vi "auto.vi"(11 "Inputs 2":T3) -> (3 "Outputs":T6)   [LabVIEW 2013]
uses:
  outputs.ctl
  drive/drive_outputs.ctl
  flinger/flinger_outputs.ctl
  <vilib>/Rock Robotics/WPI/Solenoid/WPI_SolenoidValue.ctl
  roller/roller_outputs.ctl
  catch/catch_outputs.ctl
  inputs.ctl
  drive/drive_inputs.ctl
  flinger/flinger_inputs.ctl
  roller/roller_inputs.ctl
  catch/catch_inputs.ctl
panel:
  in  "Flinger Inputs":T1
  in  "Roller Inputs":T2
  in  "Drive_inputs":T4
  in  "Inputs":T3
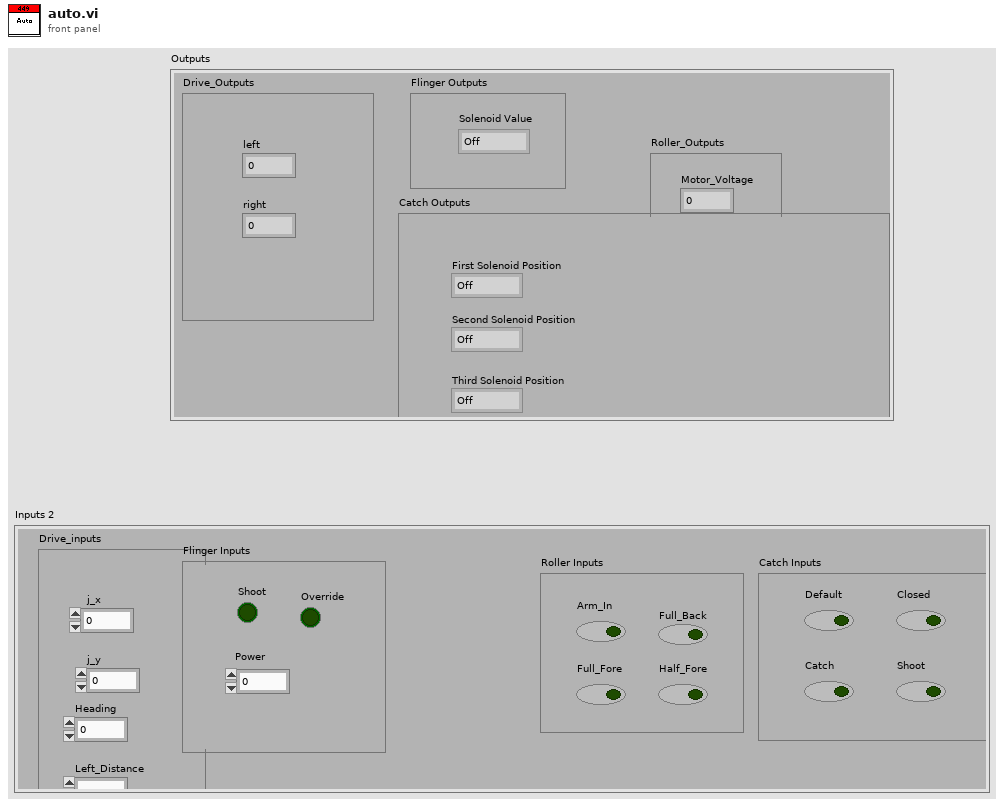
[diagram p1: front panel]
types:
  T1 = typedef "flinger_inputs.ctl" = cluster{"Shoot":bool, "Power":dbl, "Override":bool}
  T2 = typedef "roller_inputs.ctl" = cluster{"Arm_In":bool, "Full_Fore":bool, "Full_Back":bool, "Half_Fore":bool}
  T3 = typedef "inputs.ctl" = cluster{"Drive_inputs":T4, "Flinger Inputs":T1, "Roller Inputs":T2, "Catch Inputs":T5}
  T4 = typedef "drive_inputs.ctl" = cluster{"j_x":dbl, "j_y":dbl, "Heading":dbl, "Left_Distance":dbl, " Right_Distance":dbl}
  T5 = typedef "catch_inputs.ctl" = cluster{"Default":bool, "Closed":bool, "Catch":bool, "Shoot":bool}
  T6 = typedef "outputs.ctl" = cluster{"Drive_Outputs":T7, "Flinger Outputs":T8, "Roller_Outputs":T10, "Catch Outputs":T11}
  T7 = typedef "drive_outputs.ctl" = cluster{"left":dbl, "right":dbl}
  T8 = typedef "flinger_outputs.ctl" = cluster{"Solenoid Value":T9}
  T9 = typedef "WPI_SolenoidValue.ctl" = enum16{"Off", "On", "Forward", "Reverse"}
  T10 = typedef "roller_outputs.ctl" = cluster{"Sol_Position":T9, "Motor_Voltage":dbl}
  T11 = typedef "catch_outputs.ctl" = cluster{"First Solenoid Position":T9, "Second Solenoid Position":T9, "Third Solenoid Position":T9}
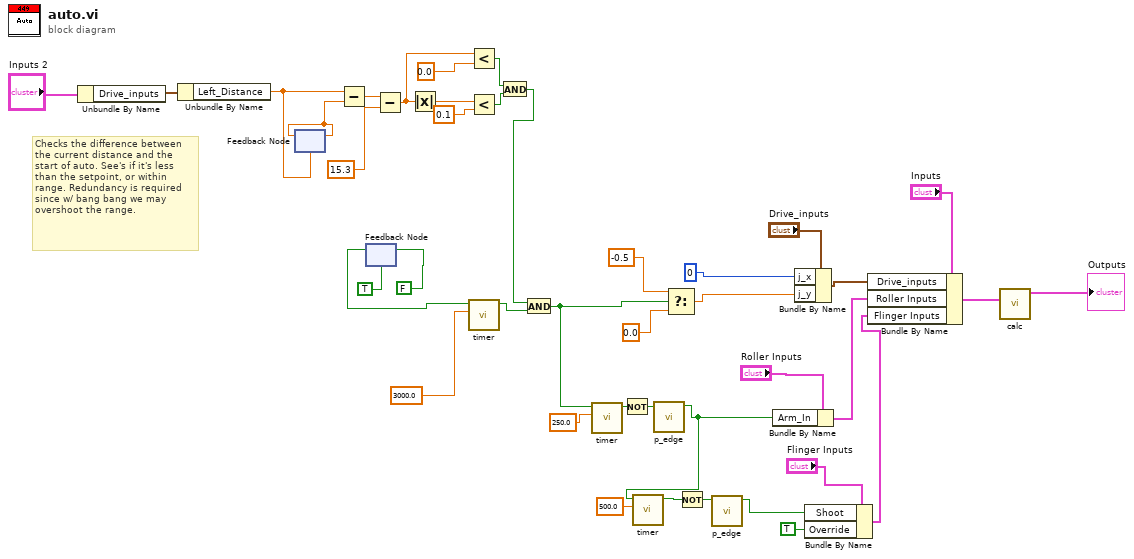
[diagram p0: block diagram]
diagram:
  # "Checks the difference between the current distance and the start of auto. See's if it's less than the setpoint, or within range. Redundancy is required since w/ bang bang we may overshoot the range."
  n1 = Unbundle By Name("Inputs 2") -> ("Drive_inputs"=w28:T4)
  n2 = Unbundle By Name(w28) -> ("Left_Distance"=w19:dbl)
  n3 = feedback #1(w19) -> (w18:dbl)
  n4 = feedback-in #1(w18) -> ()
  n5 = Subtract(x=w19, y=w18) -> (x-y=w16:dbl)
  n6 = feedback-in #2(FALSE) -> ()
  n7 = feedback #2(TRUE) -> (w31:bool)
  n8 = Subtract(x=w16, y=15.3) -> (x-y=w14:dbl)
  n9 = Absolute Value(x=w14) -> (abs(x)=w22:dbl)
  n10 = Less?(x=w14, y=0.0) -> (x < y?=w11:bool)
  n11 = Less?(x=w22, y=0.1) -> (x < y?=w10:bool)
  n12 = call "timer.vi"("Time"=3000.0, "Set"=w31) -> ("Out"=w27:bool)  [unwired: 9 in]
  n13 = And(x=w11, y=w10) -> (x .and. y?=w12:bool)
  n14 = And(x=w12, y=w27) -> (x .and. y?=w9:bool)
  n15 = call "timer.vi"("Time"=250.0, "Set"=w9) -> ("Out"=w7:bool)  [unwired: 9 in]
  n16 = Not(x=w7) -> (.not. x?=w6:bool)
  n17 = call "p_edge.vi"("In"=w6) -> ("Out"=w5:bool)  [unwired: 10 in]
  n18 = call "timer.vi"("Time"=500.0, "Set"=w5) -> ("Out"=w3:bool)  [unwired: 9 in]
  n19 = Select(t=-0.5, s=w9, f=0.0) -> (s? t:f=w35:dbl)
  n20 = Not(x=w3) -> (.not. x?=w2:bool)
  n21 = call "p_edge.vi"("In"=w2) -> ("Out"=w1:bool)  [unwired: 10 in]
  n22 = Bundle By Name(cluster="Roller Inputs", "Arm_In"=w5) -> (w20:T2)
  n23 = Bundle By Name(cluster="Drive_inputs", "j_x"=0, "j_y"=w35) -> (w38:T4)
  n24 = Bundle By Name(cluster="Flinger Inputs", "Shoot"=w1, "Override"=TRUE) -> (w25:T1)
  n25 = Bundle By Name(cluster="Inputs", "Drive_inputs"=w38, "Roller Inputs"=w20, "Flinger Inputs"=w25) -> (w40:T3)
  n26 = call "calc.vi"("Inputs"=w40) -> ("Outputs"=→"Outputs":T6)  [unwired: 10 in]
